vi "HFRR ADV v037 new software.vi"() -> ()   [LabVIEW 2025] (continued)
              disable-tunnel: "Heater On" -> [w1617 _]
              frame Enabled {
                n1486 = local read "EVENT LOG"() -> (w1618:string)
                n1487 = call "Event Log.vi"("Content"=w1617, "EVENT LOG"=w1618) -> ("EVENT LOG"=w1619:string)  [unwired: 8 in, 1 out]
                n1488 = local write "EVENT LOG"(w1619) -> ()
              }
              frame Disabled {
              }
            }
          }
        }
      }
    }
    n1489 = local read "Main Tab"() -> (w1340:T2)
    n1490 = case shown="\"About\"" w1340 {
      frame "HOME", Default {
        w1382 = T19."Enabled" ("Disabled")
        n1491 = local read "Service Password enable"() -> (w1384:bool)
        n1492 = property on="Imaging" class="Bool (strict)"("DisabledEnum"=w1382) -> ()  [unwired: 2 in, 2 out]
        n1493 = property on="Dashboard" class="Bool (strict)"("DisabledEnum"=w1382) -> ()  [unwired: 2 in, 2 out]
        n1494 = property on="Test Setup" class="Bool (strict)"("DisabledEnum"=w1382) -> ()  [unwired: 2 in, 2 out]
        n1495 = property on="Analysis" class="Bool (strict)"("DisabledEnum"=w1382) -> ()  [unwired: 2 in, 2 out]
        n1496 = property on="Home" class="Bool (strict)"("DisabledEnum"=w1382) -> ()  [unwired: 2 in, 2 out]
        n1497 = property on="Report" class="Bool (strict)"("DisabledEnum"=w1382) -> ()  [unwired: 2 in, 2 out]
        n1498 = property on="Main Dashboard Buttons" class="RadioBtnsControl (strict)"("DisabledEnum"=w1382) -> ()  [unwired: 2 in, 2 out]
        n1499 = property on="Calibration" class="Bool (strict)"("DisabledEnum"=w1382) -> ()  [unwired: 2 in, 2 out]
        n1500 = case shown="True" w1384 {
          tunnel: [T19."Disabled" ("Disabled") T19."Enabled" ("Disabled")] -> w1383
          frame False {
          }
          frame True {
          }
        }
        n1501 = property on="About" class="Bool (strict)"("DisabledEnum"=w1383) -> ()  [unwired: 2 in, 2 out]
      }
      frame "Test Setup" {
        w1389 = T19."Enabled" ("Disabled")
        n1502 = local read "Service Password enable"() -> (w1388:bool)
        n1503 = property on="Dashboard" class="Bool (strict)"("DisabledEnum"=T19."Disabled" ("Disabled")) -> ()  [unwired: 2 in, 2 out]
        n1504 = property on="Imaging" class="Bool (strict)"("DisabledEnum"=w1389) -> ()  [unwired: 2 in, 2 out]
        n1505 = property on="Analysis" class="Bool (strict)"("DisabledEnum"=w1389) -> ()  [unwired: 2 in, 2 out]
        n1506 = property on="Home" class="Bool (strict)"("DisabledEnum"=w1389) -> ()  [unwired: 2 in, 2 out]
        n1507 = property on="Report" class="Bool (strict)"("DisabledEnum"=w1389) -> ()  [unwired: 2 in, 2 out]
        n1508 = property on="Test Setup" class="Bool (strict)"("DisabledEnum"=w1389) -> ()  [unwired: 2 in, 2 out]
        n1509 = case shown="True" w1388 {
          tunnel: [T19."Disabled" ("Disabled") T19."Enabled" ("Disabled")] -> w1387
          frame False {
          }
          frame True {
          }
        }
        n1510 = property on="About" class="Bool (strict)"("DisabledEnum"=w1387) -> ()  [unwired: 2 in, 2 out]
      }
      frame "Adv Scar" {
        w1396 = T19."Enabled" ("Disabled")
        n1511 = property on="Dashboard" class="Bool (strict)"("DisabledEnum"=T19."Disabled" ("Disabled")) -> ()  [unwired: 2 in, 2 out]
        n1512 = property on="Imaging" class="Bool (strict)"("DisabledEnum"=w1396) -> ()  [unwired: 2 in, 2 out]
        n1513 = property on="Analysis" class="Bool (strict)"("DisabledEnum"=w1396) -> ()  [unwired: 2 in, 2 out]
        n1514 = property on="Home" class="Bool (strict)"("DisabledEnum"=w1396) -> ()  [unwired: 2 in, 2 out]
        n1515 = property on="Report" class="Bool (strict)"("DisabledEnum"=w1396) -> ()  [unwired: 2 in, 2 out]
        n1516 = property on="Test Setup" class="Bool (strict)"("DisabledEnum"=w1396) -> ()  [unwired: 2 in, 2 out]
        n1517 = local read "Service Password enable"() -> (w1394:bool)
        n1518 = case shown="True" w1394 {
          tunnel: [T19."Disabled" ("Disabled") T19."Enabled" ("Disabled")] -> w1393
          frame False {
          }
          frame True {
          }
        }
        n1519 = property on="About" class="Bool (strict)"("DisabledEnum"=w1393) -> ()  [unwired: 2 in, 2 out]
      }
      frame "Calibration" {
        w1399 = T19."Enabled" ("Disabled")
        n1520 = property on="Dashboard" class="Bool (strict)"("DisabledEnum"=T19."Disabled" ("Disabled")) -> ()  [unwired: 2 in, 2 out]
        n1521 = property on="Imaging" class="Bool (strict)"("DisabledEnum"=w1399) -> ()  [unwired: 2 in, 2 out]
        n1522 = property on="Analysis" class="Bool (strict)"("DisabledEnum"=w1399) -> ()  [unwired: 2 in, 2 out]
        n1523 = property on="Home" class="Bool (strict)"("DisabledEnum"=w1399) -> ()  [unwired: 2 in, 2 out]
        n1524 = property on="Report" class="Bool (strict)"("DisabledEnum"=w1399) -> ()  [unwired: 2 in, 2 out]
        n1525 = property on="Test Setup" class="Bool (strict)"("DisabledEnum"=w1399) -> ()  [unwired: 2 in, 2 out]
        n1526 = local read "Service Password enable"() -> (w1401:bool)
        n1527 = property on="Calibration" class="Bool (strict)"("DisabledEnum"=w1399) -> ()  [unwired: 2 in, 2 out]
        n1528 = case shown="True" w1401 {
          tunnel: [T19."Disabled" ("Disabled") T19."Enabled" ("Disabled")] -> w1400
          frame False {
          }
          frame True {
          }
        }
        n1529 = property on="About" class="Bool (strict)"("DisabledEnum"=w1400) -> ()  [unwired: 2 in, 2 out]
      }
      frame "Adv Scar Report" {
        w1407 = T19."Enabled" ("Disabled")
        n1530 = property on="Dashboard" class="Bool (strict)"("DisabledEnum"=T19."Disabled" ("Disabled")) -> ()  [unwired: 2 in, 2 out]
        n1531 = property on="Imaging" class="Bool (strict)"("DisabledEnum"=w1407) -> ()  [unwired: 2 in, 2 out]
        n1532 = property on="Analysis" class="Bool (strict)"("DisabledEnum"=w1407) -> ()  [unwired: 2 in, 2 out]
        n1533 = property on="Home" class="Bool (strict)"("DisabledEnum"=w1407) -> ()  [unwired: 2 in, 2 out]
        n1534 = property on="Report" class="Bool (strict)"("DisabledEnum"=w1407) -> ()  [unwired: 2 in, 2 out]
        n1535 = property on="Test Setup" class="Bool (strict)"("DisabledEnum"=w1407) -> ()  [unwired: 2 in, 2 out]
        n1536 = local read "Service Password enable"() -> (w1406:bool)
        n1537 = case shown="True" w1406 {
          tunnel: [T19."Disabled" ("Disabled") T19."Enabled" ("Disabled")] -> w1405
          frame False {
          }
          frame True {
          }
        }
        n1538 = property on="About" class="Bool (strict)"("DisabledEnum"=w1405) -> ()  [unwired: 2 in, 2 out]
      }
      frame "Compare Files" {
        w1413 = T19."Enabled" ("Disabled")
        n1539 = local read "Service Password enable"() -> (w1412:bool)
        n1540 = property on="Dashboard" class="Bool (strict)"("DisabledEnum"=T19."Disabled" ("Disabled")) -> ()  [unwired: 2 in, 2 out]
        n1541 = property on="Imaging" class="Bool (strict)"("DisabledEnum"=w1413) -> ()  [unwired: 2 in, 2 out]
        n1542 = property on="Analysis" class="Bool (strict)"("DisabledEnum"=w1413) -> ()  [unwired: 2 in, 2 out]
        n1543 = property on="Home" class="Bool (strict)"("DisabledEnum"=w1413) -> ()  [unwired: 2 in, 2 out]
        n1544 = property on="Report" class="Bool (strict)"("DisabledEnum"=w1413) -> ()  [unwired: 2 in, 2 out]
        n1545 = property on="Test Setup" class="Bool (strict)"("DisabledEnum"=w1413) -> ()  [unwired: 2 in, 2 out]
        n1546 = case shown="True" w1412 {
          tunnel: [T19."Disabled" ("Disabled") T19."Enabled" ("Disabled")] -> w1411
          frame False {
          }
          frame True {
          }
        }
        n1547 = property on="About" class="Bool (strict)"("DisabledEnum"=w1411) -> ()  [unwired: 2 in, 2 out]
      }
      frame "Acquire" {
        n1548 = local read "Service Password enable"() -> (w1418:bool)
        n1549 = property on="Test Setup" class="Bool (strict)"("DisabledEnum"=T19."Disabled" ("Disabled")) -> ()  [unwired: 2 in, 2 out]
        n1550 = local read "Auto Start Test"() -> (w1420:bool)
        n1551 = local read "RUN"() -> (w1422:bool)
        n1552 = case shown="True" w1418 {
          tunnel: [T19."Disabled" ("Disabled") T19."Enabled" ("Disabled")] -> w1419
          frame False {
          }
          frame True {
          }
        }
        n1553 = Or(x=w1422, y=w1420) -> (x .or. y?=w1421:bool)
        n1554 = case shown="True" w1421 {
          tunnel: [T19."Enabled" ("Disabled") T19."Disabled" ("Disabled")] -> w1417
          frame False {
          }
          frame True {
          }
        }
        n1555 = property on="About" class="Bool (strict)"("DisabledEnum"=w1419) -> ()  [unwired: 2 in, 2 out]
        n1556 = property on="Imaging" class="Bool (strict)"("DisabledEnum"=w1417) -> ()  [unwired: 2 in, 2 out]
        n1557 = property on="Dashboard" class="Bool (strict)"("DisabledEnum"=w1417) -> ()  [unwired: 2 in, 2 out]
        n1558 = property on="Analysis" class="Bool (strict)"("DisabledEnum"=w1417) -> ()  [unwired: 2 in, 2 out]
        n1559 = property on="Home" class="Bool (strict)"("DisabledEnum"=w1417) -> ()  [unwired: 2 in, 2 out]
        n1560 = property on="Report" class="Bool (strict)"("DisabledEnum"=w1417) -> ()  [unwired: 2 in, 2 out]
        n1561 = property on="Calibration" class="Bool (strict)"("DisabledEnum"=w1417) -> ()  [unwired: 2 in, 2 out]
      }
      frame "About" {
        n1562 = local read "FILE"() -> (w1436:string)
        n1563 = local read "TEST FILE NAM,E SAVED"() -> (w1429:bool)
        n1564 = call <vilib>:"Trim Whitespace.vi"("string"=w1436) -> ("trimmed string"=w1435:string)  [unwired: 1 in]
        n1565 = local read "Auto Start Test"() -> (w1439:bool)
        n1566 = String Length(string=w1435) -> (length=w1434:i32)
        n1567 = Greater?(x=w1434, y=1) -> (0:w1431:bool)
        n1568 = And(x=w1431, y=w1429) -> (x .and. y?=w1430:bool)
        n1569 = local read "RUN"() -> (w1441:bool)
        n1570 = case shown="True" w1430 {
          tunnel: [T19."Disabled" ("Disabled") T19."Enabled" ("Disabled")] -> w1432
          frame False {
          }
          frame True {
          }
        }
        n1571 = Or(x=w1441, y=w1439) -> (x .or. y?=w1440:bool)
        n1572 = property on="About" class="Bool (strict)"("DisabledEnum"=T19."Enabled" ("Disabled")) -> ()  [unwired: 2 in, 2 out]
        n1573 = case shown="False" w1440 {
          tunnel: [T19."Enabled" ("Disabled") T19."Disabled" ("Disabled")] -> w1438
          frame False {
          }
          frame True {
          }
        }
        n1574 = property on="Dashboard" class="Bool (strict)"("DisabledEnum"=w1432) -> ()  [unwired: 2 in, 2 out]
        n1575 = property on="Test Setup" class="Bool (strict)"("DisabledEnum"=T19."Disabled" ("Disabled")) -> ()  [unwired: 2 in, 2 out]
        n1576 = property on="Imaging" class="Bool (strict)"("DisabledEnum"=w1438) -> ()  [unwired: 2 in, 2 out]
        n1577 = property on="Analysis" class="Bool (strict)"("DisabledEnum"=w1438) -> ()  [unwired: 2 in, 2 out]
        n1578 = property on="Home" class="Bool (strict)"("DisabledEnum"=w1438) -> ()  [unwired: 2 in, 2 out]
        n1579 = property on="Report" class="Bool (strict)"("DisabledEnum"=w1438) -> ()  [unwired: 2 in, 2 out]
      }
    }
    n1580 = local read "Quit"() -> (w1366:bool)
    "Single" <- "Single - Graph"
  }
  n1581 = disable-structure shown="Disabled" {
    disable-tunnel: [w1719 _] -> w42
    disable-tunnel: _ -> [w1718 _]
    frame Disabled {
      n1582 = while {
        tunnel: w1718 -> [_]
        tunnel: [w1720] -> w1719
        tunnel: [w1721] -> _
        i -> [w1721]
        stop <- w1720 stop-if-true
        w1737 = u16 10 items=["1.0"=10, "1.5"=15, "2.0"=20] ("stop bits (10: 1 bit)")
        n1583 = Wait (ms)(milliseconds to wait=u32 10) -> ()  [unwired: 1 out]
        n1584 = call-poly "VISA Configure Serial Port"("VISA resource name"=refnum<visa-resource-name> "ASRL1::INSTR" ("COM PORT"), "timeout (10sec)"=u32 10, "baud rate (9600)"=u32 57600, "data bits (8)"=u16 8, "stop bits (10: 1 bit)"=w1737) -> ("VISA resource name out"=w1723:refnum<visa-resource-name>, "error out"=w1732:errorcluster)  [unwired: 9 in]
        n1585 = VISA Read(VISA resource name=w1723, byte count=u32 2 ("byte count (0)")) -> (read buffer=w1731:string)  [unwired: 1 in, 3 out]
        n1586 = String Subset(string=w1731, offset (0)=0, length (rest)=2 ("length (rest)")) -> (substring=w1730:string)
        n1587 = Match Pattern(string=w1730, regular expression="<>") -> (offset past match=w1727:i32)  [unwired: 1 in, 3 out]
        n1588 = Greater Or Equal?(x=w1727, y=0) -> (x >= y?=w1722:bool)
        n1589 = case shown="True" w1722 {
          tunnel: w1723 -> [_ w1741]
          tunnel: w1732 -> [_ w1740]
          frame False {
          }
          frame True {
            n1590 = VISA Read(VISA resource name=w1741, byte count=u32 32 ("byte count (0)"), error in (no error)=w1740) -> (read buffer=w1739:string)  [unwired: 3 out]
            n1591 = String Subset(string=w1739, offset (0)=0, length (rest)=8 ("length (rest)")) -> (substring=w1743:string)
            n1592 = String Subset(string=w1739, offset (0)=8, length (rest)=8 ("length (rest)")) -> (substring=w1744:string)
            n1593 = Decimal String To Number(string=w1744) -> (number=w1751:i32)  [unwired: 2 in, 1 out]
            n1594 = Decimal String To Number(string=w1743) -> (number=w1747:i32)  [unwired: 2 in, 1 out]
            n1595 = Divide(x=w1751, y=10000) -> ()  [unwired: 1 out]
            n1596 = Divide(x=w1747, y=1000000) -> ()  [unwired: 1 out]
          }
        }
        n1597 = local read "Quit"() -> (w1720:bool)
      }
    }
    frame Enabled {
    }
  }
  n1598 = Tick Count (ms)() -> (millisecond timer value=w4:u32)
  n1599 = while {
    shift-right: [w1797] -> _
    shift-left: w6 -> [w1801]
    shift-right: [w1796] -> _
    shift-left: w5 -> [w1800]
    shift-right: [w1795] -> _
    shift-left: w6 -> [w1799]
    shift-right: [w1794] -> _
    shift-left: w5 -> [w1798]
    shift-right: [w1792] -> _
    shift-left: w4 -> [w1793]
    shift-right: [w1789] -> _
    shift-left: w3 -> [w1790]
    shift-right: [w1788] -> _
    shift-left: w3 -> [w1791]
    shift-right: [w1781] -> _
    shift-left: w3 -> [w1787]
    shift-right: [w1780] -> _
    shift-left: w3 -> [w1786]
    shift-right: [w1779] -> _
    shift-left: w3 -> [w1785]
    shift-right: [w1778] -> _
    shift-left: w3 -> [w1784]
    shift-right: [w1777] -> _
    shift-left: w3 -> [w1783]
    shift-right: [w1776] -> _
    shift-left: w3 -> [w1782]
    shift-right: [w1775] -> _
    shift-left: w3 -> [w1769]
    shift-right: [w1774] -> _
    shift-left: w3 -> [w1768]
    shift-right: [w1773] -> _
    shift-left: w3 -> [w1767]
    shift-right: [w1772] -> _
    shift-left: w3 -> [w1766]
    shift-right: [w1771] -> _
    shift-left: w3 -> [w1765]
    shift-right: [w1770] -> _
    shift-left: w3 -> [w1764]
    shift-right: [w1755] -> _
    shift-left: w3 -> [w1758]
    shift-right: [w1754] -> _
    shift-left: w3 -> [w1757]
    shift-right: [w1753] -> _
    shift-left: w3 -> [w1756]
    stop <- w1803 stop-if-true
    n1600 = local read "Read UNO"() -> (w1762:string)
    n1601 = local read "Error  2"() -> (w1802:errorcluster)
    n1602 = String Length(string=w1762) -> (length=w1761:i32)
    n1603 = call <vilib>:"Trim Whitespace.vi"("string"=w1762) -> ("trimmed string"=w1763:string)  [unwired: 1 in]
    n1604 = Greater Or Equal?(x=w1761, y=23) -> (x >= y?=w1759:bool)
    n1605 = case shown="No Error" w1802 {
      tunnel: w1801 -> [w1849 w1945]
      tunnel: w1800 -> [w1848 w1944]
      tunnel: w1799 -> [w1847 w1943]
      tunnel: w1798 -> [w1846 w1942]
      tunnel: [w1845 w1945] -> w1797
      tunnel: [w1844 w1944] -> w1796
      tunnel: [w1843 w1943] -> w1795
      tunnel: [w1842 w1942] -> w1794
      tunnel: w1793 -> [w1841 w1941]
      tunnel: [w1840 w1941] -> w1792
      tunnel: w1790 -> [w1839 w1940]
      tunnel: w1791 -> [w1838 w1939]
      tunnel: [w1837 w1940] -> w1789
      tunnel: [w1836 w1939] -> w1788
      tunnel: w1787 -> [w1835 w1938]
      tunnel: w1786 -> [w1834 w1937]
      tunnel: w1785 -> [w1833 w1936]
      tunnel: w1784 -> [w1832 w1935]
      tunnel: w1783 -> [w1831 w1934]
      tunnel: w1782 -> [w1830 w1933]
      tunnel: [w1829 w1938] -> w1781
      tunnel: [w1828 w1937] -> w1780
      tunnel: [w1827 w1936] -> w1779
      tunnel: [w1826 w1935] -> w1778
      tunnel: [w1825 w1934] -> w1777
      tunnel: [w1824 w1933] -> w1776
      tunnel: w1769 -> [w1823 w1932]
      tunnel: [w1822 w1932] -> w1775
      tunnel: [w1821 w1928] -> w1774
      tunnel: [w1820 w1927] -> w1773
      tunnel: [w1819 w1931] -> w1772
      tunnel: [w1818 w1930] -> w1771
      tunnel: [w1817 w1929] -> w1770
      tunnel: w1768 -> [w1816 w1931]
      tunnel: w1767 -> [w1815 w1930]
      tunnel: w1766 -> [w1814 w1929]
      tunnel: w1765 -> [w1813 w1928]
      tunnel: w1764 -> [w1812 w1927]
      tunnel: w1763 -> [w1811 _]
      tunnel: w1759 -> [w1810 _]
      tunnel: w1758 -> [w1809 w1926]
      tunnel: w1757 -> [w1808 w1925]
      tunnel: w1756 -> [w1807 w1924]
      tunnel: [w1806 w1926] -> w1755
      tunnel: [w1805 w1925] -> w1754
      tunnel: [w1804 w1924] -> w1753
      frame No Error {
        n1606 = case shown="True" w1810 {
          tunnel: w1849 -> [w1865 w1917]
          tunnel: w1848 -> [w1864 w1916]
          tunnel: w1847 -> [w1863 w1915]
          tunnel: w1846 -> [w1862 w1914]
          tunnel: [w1865 w1913] -> w1845
          tunnel: [w1864 w1912] -> w1844
          tunnel: [w1863 w1911] -> w1843
          tunnel: [w1862 w1910] -> w1842
          tunnel: w1841 -> [w1861 w1908]
          tunnel: [w1861 w1907] -> w1840
          tunnel: w1839 -> [w1860 w1906]
          tunnel: w1838 -> [w1859 w1905]
          tunnel: [w1860 w1904] -> w1837
          tunnel: [w1859 w1903] -> w1836
          tunnel: w1835 -> [w1858 w1902]
          tunnel: w1834 -> [w1857 w1901]
          tunnel: w1833 -> [w1856 w1900]
          tunnel: w1832 -> [w1855 w1899]
          tunnel: w1831 -> [w1854 w1898]
          tunnel: w1830 -> [w1853 w1897]
          tunnel: [w1858 w1896] -> w1829
          tunnel: [w1857 w1895] -> w1828
          tunnel: [w1856 w1894] -> w1827
          tunnel: [w1855 w1893] -> w1826
          tunnel: [w1854 w1892] -> w1825
          tunnel: [w1853 w1891] -> w1824
          tunnel: w1823 -> [w1871 w1890]
          tunnel: [w1871 w1889] -> w1822
          tunnel: [w1868 w1888] -> w1821
          tunnel: [w1867 w1887] -> w1820
          tunnel: [w1870 w1886] -> w1819
          tunnel: [w1866 w1885] -> w1818
          tunnel: [w1869 w1884] -> w1817
          tunnel: w1816 -> [w1870 w1883]
          tunnel: w1815 -> [w1869 w1882]
          tunnel: w1814 -> [w1868 w1881]
          tunnel: w1813 -> [w1867 w1880]
          tunnel: w1812 -> [w1866 w1879]
          tunnel: w1811 -> [_ w1878]
          tunnel: w1809 -> [w1852 w1877]
          tunnel: w1808 -> [w1851 w1876]
          tunnel: w1807 -> [w1850 w1875]
          tunnel: [w1852 w1874] -> w1806
          tunnel: [w1851 w1873] -> w1805
          tunnel: [w1850 w1872] -> w1804
          frame False {
          }
          frame True {
            n1607 = Tick Count (ms)() -> (millisecond timer value=w1909:u32)
            n1608 = String To Byte Array(string=w1878) -> (unsigned byte array=w1922:u8[])
            n1609 = Array Size(array=w1922) -> (size(s)=w1921:i32)
            n1610 = formula code="// --- INTERNAL VARIABLE DECLARATIONS ---\nint i = 0;\nint k = 0;\nint start_idx = -1;\nint end_idx = -1;\nint phase = 0;\nint sign0 = 1;\nint sign1 = 1;\nint ch0_val = 0;   \nint ch1_val = 0;   \nfloat ch0_raw = 0.0;\nfloat ch1_raw = 0.0;\nfloat temp0 = 0.0;\nfloat temp1 = 0.0;\nfloat ch0_clean = 0.0;\nfloat ch1_clean = 0.0;\n\nint valid_samples = 0; // FIX: Track if we actually parsed new data this window\nfloat max_allowed_bits = 8388607.0; // FIX: Change this to match your ADC max value\n\n// Temporal intermediate variables for calculation smoothing\nfloat raw_p2p_v = 0.0;\nfloat raw_friction = 0.0;\nfloat raw_cof = 0.0;\n\n// Temporal intermediate variables for Piezo voltage translations\nfloat piezo_min_v = 0.0;\nfloat piezo_max_v = 0.0;\n\n// Initialize output variables to current shift register states right away\nout_LVDT_Min_V = in_LVDT_Min_V;\nout_LVDT_Max_V = in_LVDT_Max_V;\nout_LVDT_P2P_V = in_LVDT_P2P_V;\nout_Piezo_P2P = in_Piezo_P2P;\nout_Friction_N = in_Friction_N;\nout_COF = in_COF;\nwindow_ready = 0;\n\n// --- STEP 1: PARSE EVERY STRING IN THE BYTE ARRAY ---\nif (array_size > 2) {\n    for (i = 0; i < array_size - 1; i++) {\n        if (raw_bytes[i] == 42) { // '*' character detected\n            start_idx = i;\n        }\n        \n        // Match standard delimiter sequence \";&\" or end window character\n        if (raw_bytes[i] == 59 && raw_bytes[i+1] == 38 && start_idx != -1) { \n            end_idx = i;\n            ch0_val = 0;\n            ch1_val = 0;\n            sign0 = 1;\n            sign1 = 1;\n            phase = 0; \n\n            for (k = start_idx + 1; k < end_idx; k++) {\n                if (raw_bytes[k] == 45) { // '-' sign\n                    if (phase == 0) sign0 = -1;\n                    else sign1 = -1;\n                }\n                else if (raw_bytes[k] == 43) { // '+' sign\n                    if (phase == 0) sign0 = 1;\n                    else sign1 = 1;\n                }\n                else if (raw_bytes[k] == 59) { // ';' delimiter\n                    phase = 1; \n                }\n                else if (raw_bytes[k] >= 48 && raw_bytes[k] <= 57) { // Numeric ASCII digits\n                    if (phase == 0) {\n                        ch0_val = (ch0_val * 10) + (raw_bytes[k] - 48);\n                    } else {\n                        ch1_val = (ch1_val * 10) + (raw_bytes[k] - 48);\n                    }\n                }\n            }\n\n            // Implicit type conversion\n            ch0_raw = ch0_val * sign0 * 1.0;\n            ch1_raw = ch1_val * sign1 * 1.0;\n\n            // FIX: Sanity check / Hard-clamping to catch sudden massive ASCII noise spikes\n            if (ch0_raw > max_allowed_bits)  ch0_raw = max_allowed_bits;\n            if (ch0_raw < -max_allowed_bits) ch0_raw = -max_allowed_bits;\n            if (ch1_raw > max_allowed_bits)  ch1_raw = max_allowed_bits;\n            if (ch1_raw < -max_allowed_bits) ch1_raw = -max_allowed_bits;\n\n            // --- STEP 2: 3-SAMPLE MEDIAN FILTER ---\n            m0_2 = m0_1; m0_1 = m0_0; m0_0 = ch0_raw;\n            float s0_0 = m0_0; float s0_1 = m0_1; float s0_2 = m0_2;\n            if (s0_0 > s0_1) { temp0 = s0_0; s0_0 = s0_1; s0_1 = temp0; }\n            if (s0_1 > s0_2) { temp0 = s0_1; s0_1 = s0_2; s0_2 = temp0; }\n            if (s0_0 > s0_1) { temp0 = s0_0; s0_0 = s0_1; s0_1 = temp0; }\n            ch0_clean = s0_1;\n\n            m1_2 = m1_1; m1_1 = m1_0; m1_0 = ch1_raw;\n            float s1_0 = m1_0; float s1_1 = m1_1; float s1_2 = m1_2;\n            if (s1_0 > s1_1) { temp1 = s1_0; s1_0 = s1_1; s1_1 = temp1; }\n            if (s1_1 > s1_2) { temp1 = s1_1; s1_1 = s1_2; s1_2 = temp1; }\n            if (s1_0 > s1_1) { temp1 = s1_0; s1_0 = s1_1; s1_1 = temp1; }\n            ch1_clean = s1_1;\n\n            // --- STEP 3: EXPONENTIAL FILTER (STREAM LEVEL) ---\n            if (ch0_filt == 0.0) ch0_filt = ch0_clean;\n            if (ch1_filt == 0.0) ch1_filt = ch1_clean;\n\n            ch0_filt = ch0_filt + (ch0_clean - ch0_filt) * 0.125;\n            ch1_filt = ch1_filt + (ch1_clean - ch1_filt) * 0.125;\n\n            // --- STEP 4: MIN/MAX WINDOW CONTINUOUS ACCUMULATION ---\n            if (ch0_filt > max_ch0) max_ch0 = ch0_filt;\n            if (ch0_filt < min_ch0) min_ch0 = ch0_filt;\n            if (ch1_filt > max_ch1) max_ch1 = ch1_filt;\n            if (ch1_filt < min_ch1) min_ch1 = ch1_filt;\n\n            valid_samples++; // FIX: Successfully parsed and accumulated a clean point\n            start_idx = -1; \n        }\n    }\n}\n\n// --- STEP 5: WINDOW EVALUATION ENGINE ---\n// FIX: Condition updated to verify that valid samples exist for both channels\nif (((current_time_ms - start_time_ms) >= 50) && (valid_samples > 0) && (min_ch0 < 9000000.0) && (min_ch1 < 9000000.0)) {\n    window_ready = 1;\n\n    // Linear Bit-to-Voltage Transformations (LVDT - Channel 0)\n    out_LVDT_Min_V = (min_ch0 * VREF) / 8388607.0;\n    out_LVDT_Max_V = (max_ch0 * VREF) / 8388607.0;\n    raw_p2p_v = out_LVDT_Max_V - out_LVDT_Min_V;\n\n    // Linear Bit-to-Voltage Transformations (Piezo - Channel 1)\n    piezo_min_v = (min_ch1 * VREF) / 8388607.0;\n    piezo_max_v = (max_ch1 * VREF) / 8388607.0;\n    \n    // Assign Peak-to-Peak Voltage directly to output indicator (Matches Python logic)\n    out_Piezo_P2P = piezo_max_v - piezo_min_v;\n    \n    // Force scaling calculations using Voltage delta * Newtons/Volt Factor\n    raw_friction = out_Piezo_P2P * PIEZO_CAL_FACTOR + 0.44528;\n    raw_cof = raw_friction / NORMAL_FORCE;\n\n    // --- STEP 6: OUTPUT METRIC SMOOTHING (Low-Pass Filter Alpha = 0.05) ---\n    // Seed initial historical metrics if first loop iteration\n    if (hist_LVDT_P2P == 0.0) hist_LVDT_P2P = raw_p2p_v;\n    if (hist_Friction == 0.0) hist_Friction = raw_friction;\n    if (hist_COF == 0.0)      hist_COF = raw_cof;\n\n    // Apply exponential output dampening\n    hist_LVDT_P2P = hist_LVDT_P2P + (raw_p2p_v - hist_LVDT_P2P) * 0.05;\n    hist_Friction = hist_Friction + (raw_friction - hist_Friction) * 0.05; // Note: Can drop to 0.02 for more aggressive damping\n    hist_COF      = hist_COF + (raw_cof - hist_COF) * 0.05;\n\n    // Direct smoothed parameters out to UI Indicators\n    out_LVDT_P2P_V = hist_LVDT_P2P;\n    out_Friction_N = hist_Friction;\n    out_COF        = hist_COF;\n\n    // Reset tracking targets to extreme boundaries safely\n    min_ch0 = 9999999.0;\n    max_ch0 = -9999999.0;\n    min_ch1 = 9999999.0;\n    max_ch1 = -9999999.0;\n\n    valid_samples = 0; // FIX: Reset counter for next time frame\n    start_time_ms = current_time_ms;\n}"("raw_bytes"=w1922, "array_size"=w1921, "VREF"="VREF", "PIEZO_CAL_FACTOR"="PIEZO_CAL_FACTOR", "NORMAL_FORCE"="NORMAL_FORCE", "min_ch0"=w1917, "max_ch0"=w1916, "min_ch1"=w1915, "max_ch1"=w1914, "current_time_ms"=w1909, "start_time_ms"=w1908, "ch0_filt"=w1906, "ch1_filt"=w1905, "m0_0"=w1902, "m0_1"=w1901, "m0_2"=w1900, "m1_0"=w1899, "m1_1"=w1898, "m1_2"=w1897, "in_LVDT_Min_V"=w1890, "in_LVDT_Max_V"=w1883, "in_LVDT_P2P_V"=w1882, "in_Piezo_P2P"=w1881, "in_Friction_N"=w1880, "in_COF"=w1879, "hist_LVDT_P2P"=w1877, "hist_Friction"=w1876, "hist_COF"=w1875) -> ("window_ready"=→"Valid_data":dbl, "out_LVDT_Min_V"=w1889:dbl, "out_LVDT_Max_V"=w1888:dbl, "out_LVDT_P2P_V"=w1887:dbl, "out_Piezo_P2P"=w1886:dbl, "out_Friction_N"=w1885:dbl, "out_COF"=w1884:dbl, "min_ch0"=w1913:dbl, "max_ch0"=w1912:dbl, "min_ch1"=w1911:dbl, "max_ch1"=w1910:dbl, "start_time_ms"=w1907:u32, "ch0_filt"=w1904:dbl, "ch1_filt"=w1903:dbl, "m0_0"=w1896:dbl, "m0_1"=w1895:dbl, "m0_2"=w1894:dbl, "m1_0"=w1893:dbl, "m1_1"=w1892:dbl, "m1_2"=w1891:dbl, "hist_LVDT_P2P"=w1874:dbl, "hist_Friction"=w1873:dbl, "hist_COF"=w1872:dbl)
            "LVDT MIN" <- w1889
            "LVDT MAX" <- w1888
            "LVDT Peak" <- w1887
            "pizo raw" <- w1886
            "cof" <- w1884
            "Frictioin Force Raw" <- w1885
          }
        }
      }
      frame Error {
      }
    }
    n1611 = local read "Quit"() -> (w1803:bool)
  }
  n1612 = disable-structure shown="Disabled" {
    disable-tunnel: errorcluster {"status"=TRUE, "code"=0, "source"="Init"} ("error IO") -> [w1948 _]
    disable-tunnel: [w1946 _] -> w45
    frame Disabled {
      n1613 = while {
        shift-right: [w1964] -> w1950
        shift-left: _ -> [w1955]
        shift-right: [w1963] -> w1949
        shift-left: w1948 -> [w1957]
        tunnel: [w1952] -> w1946
        tunnel: [w1962] -> _
        i -> [w1962]
        stop <- w1952 stop-if-true
        n1614 = local read "Port 1a"() -> (w1958:bool)
        n1615 = local read "Port 3"() -> (w1959:bool)
        n1616 = local read "Com Port 1"() -> (w1956:refnum<visa-resource-name>)
        n1617 = Or(x=w1959, y=w1958) -> (x .or. y?=w1961:bool)
        n1618 = Unbundle(w1957) -> ("status"=→"Port 3":bool)  [unwired: 2 out]
        n1619 = Not Equal?(x=w1956, y=w1955) -> (x != y?=w1953:bool)
        n1620 = case shown="True" w1961 {
          frame False {
            w1967 = TRUE ("Visible")
            n1621 = property on="Port 1a" class="Bool (strict)"("Visible"=w1967) -> ()  [unwired: 2 in, 2 out]
            n1622 = property on="Port 3" class="Bool (strict)"("Visible"=w1967) -> ()  [unwired: 2 in, 2 out]
          }
          frame True {
            w1968 = TRUE ("Visible")
            n1623 = property on="Port 1a" class="Bool (strict)"("Visible"=w1968) -> ()  [unwired: 2 in, 2 out]
            n1624 = property on="Port 3" class="Bool (strict)"("Visible"=w1968) -> ()  [unwired: 2 in, 2 out]
          }
        }
        n1625 = Wait (ms)(milliseconds to wait=u32 40) -> ()  [unwired: 1 out]
        n1626 = case shown="True" w1953 {
          tunnel: [w1965 errorcluster {"status"=TRUE, "code"=0, "source"="Init"} ("error out")] -> w1954
          tunnel: w1957 -> [w1965 _]
          frame False {
          }
          frame True {
          }
        }
        n1627 = case shown="Error" w1954 {
          selector: w1954 -> [w1975 w1993]
          tunnel: [w1978 w1997] -> w1964
          tunnel: [w1977 w1991] -> w1963
          tunnel: w1955 -> [w1976 w1995]
          frame No Error {
            n1628 = property class="Instr"(reference=w1976, error in=w1975) -> (reference out=w1973:refnum<visa-resource-name>, error out=w1974:errorcluster, "Serial Settings:Number of Bytes at Serial Port"=w1970:u32)
            n1629 = Greater?(x=w1970, y=u32 5) -> (0:w1969:bool)
            n1630 = Not(x=w1969) -> (.not. x?=→"Port 1a":bool)
            n1631 = while {
              tunnel: [w1986] -> w1977
              tunnel: [w1985] -> w1978
              tunnel: w1974 -> [w1984]
              tunnel: w1973 -> [w1983]
              stop <- TRUE stop-if-true
              n1632 = property class="Instr" props=["Serial Settings:Number of Bytes at Serial Port"](reference=w1983, error in=w1984) -> (reference out=w1988:refnum<visa-resource-name>, error out=w1987:errorcluster)  [unwired: 1 out]
              n1633 = VISA Read(VISA resource name=w1988, byte count=u32 50, error in (no error)=w1987) -> (VISA resource name out=w1985:refnum<visa-resource-name>, read buffer=w1980:string, error out=w1986:errorcluster)  [unwired: 1 out]
              n1634 = Wait (ms)(milliseconds to wait=u32 5) -> ()  [unwired: 1 out]
            }
          }
          frame Error {
            w2003 = u16 0 items=["None", "XON/XOFF", "RTS/CTS", "XON/XOFF & RTS/CTS", "DTR/DSR", "XON/XOFF & DTR/DSR"] ("flow control (0:none)  2")
            w2001 = u16 10 items=["1.0"=10, "1.5"=15, "2.0"=20] ("stop bits 2")
            w1999 = u16 0 items=["None", "Odd", "Even", "Mark", "Space"] ("parity 2")
            w2000 = u32 10000  # timeout (10sec)
            n1635 = VISA Close(VISA resource name=w1995, error in (no error)=w1993) -> (error out=w1996:errorcluster)
            n1636 = local write "Port 1a"(FALSE ("Port 1a")) -> ()
            n1637 = local read "Com Port 1"() -> (w1990:refnum<visa-resource-name>)
            n1638 = call <vilib>:"Clear Errors.vi"("error in (no error)"=w1996) -> ("error out"=w1994:errorcluster)  [unwired: 5 in, 1 out]
            n1639 = call-poly "VISA Configure Serial Port"("VISA resource name"=w1990, "timeout (10sec)"=w2000, "baud rate (9600)"=u32 250000 ("baud rate  2"), "data bits (8)"=u16 8 ("data bits  2"), "parity (0:none)"=w1999, "error in (no error)"=w1994, "stop bits (10: 1 bit)"=w2001, "flow control (0:none)"=w2003) -> ("VISA resource name out"=w2004:refnum<visa-resource-name>, "error out"=w2005:errorcluster)  [unwired: 6 in]
            n1640 = flat-sequence {
              tunnel: w2004 -> [w2007]
              tunnel: w2005 -> [w2006]
              tunnel: [w2007] -> w1997
              tunnel: [w2006] -> w1991
              frame #0 {
                n1641 = Wait (ms)(milliseconds to wait=u32 50) -> ()  [unwired: 1 out]
              }
            }
            "Residual Uno" <- ""
          }
        }
        n1642 = local read "Quit"() -> (w1952:bool)
        "Error Uno" <- w1957
      }
      n1643 = VISA Close(VISA resource name=w1950, error in (no error)=w1949) -> (error out=w1947:errorcluster)
      n1644 = call <vilib>:"Clear Errors.vi"("error in (no error)"=w1947) -> ()  [unwired: 5 in, 2 out]
    }
    frame Enabled {
    }
  }
  n1645 = while {
    stop <- w2018 stop-if-true
    # "V0OLTAGE TO STROKE (peice vise calibration)"
    n1646 = local read "LVDT MIN"() -> (w2010:dbl)
    n1647 = local read "LVDT Peak"() -> (w2009:dbl)
    n1648 = Wait (ms)(milliseconds to wait=u32 10) -> ()  [unwired: 1 out]
    n1649 = formula code="// Dynamic Parameterized Linear Interpolation Node\n// Inputs: vpp_val, voltages (Array), distances (Array)\n// Outputs: stroke\n\nint i = 0;\nint segments = 11; // 12 points make 11 interpolation segments\n\n// 1. Lower Boundary Clamp\nif (vpp_val <= voltages[0]) {\n    stroke = distances[0];\n}\n// 2. Upper Boundary Clamp\nelse if (vpp_val >= voltages[segments]) {\n    stroke = distances[segments];\n}\n// 3. Dynamic Segment Search Loop\nelse {\n    stroke = distances[0]; // Fallback baseline\n    for (i = 0; i < segments; i++) {\n        if (vpp_val >= voltages[i] && vpp_val <= voltages[i+1]) {\n            // Standard linear interpolation formula using array lookups\n            stroke = distances[i] + (vpp_val - voltages[i]) * (distances[i+1] - distances[i]) / (voltages[i+1] - voltages[i]);\n            break; // Segment found, safely exit the loop\n        }\n    }\n}"("vpp_val"=w2009, "voltages"="calibration values", "distances"="STROKE") -> ("stroke"=→"LVDT STROKE":dbl)
    n1650 = local read "Calibration Tare Value"() -> (w2014:dbl)
    n1651 = local read "Calibration Tare"() -> (w2012:bool)
    n1652 = Subtract(x=w2010, y=w2014) -> (x-y=→"LVDT STROKE  Calibration":dbl)
    n1653 = case shown="True" w2012 {
      selector: w2012 -> [_ w2020]
      tunnel: w2010 -> [_ w2021]
      frame False {
      }
      frame True {
        n1654 = Not(x=w2020) -> (.not. x?=w2019:bool)
        n1655 = local write "Calibration Tare"(w2019) -> ()
        "Calibration Tare Value" <- w2021
      }
    }
    n1656 = local read "Quit"() -> (w2018:bool)
  }
  n1657 = while {
    stop <- w2044 stop-if-true
    n1658 = local read "Due read"() -> (w2042:string)
    n1659 = call <vilib>:"High Resolution Polling Wait.vi"("seconds to wait"=0.02) -> ()  [unwired: 10 in, 1 out]
    n1660 = local read "Frictioin Force Raw"() -> (w2024:dbl)
    n1661 = Spreadsheet String To Array(delimiter (Tab)=";", format string="", spreadsheet string=w2042, array type (2D Dbl)=string[] []) -> (array=w2039:string[])
    n1662 = Fract/Exp String To Number(string=w2039) -> (number=w2038:dbl[])  [unwired: 3 in, 1 out]
    n1663 = call <vilib>:"Median Filter PtByPt.vi"("rank"=2, "x"=w2024) -> ("Filtered x"=→"Friction":dbl)  [unwired: 2 in, 1 out]
    n1664 = Index Array(array=w2038) -> (element #1=→"Sample Temperature":dbl, element #2=→"Target Sample Temperature":dbl, element #3=→"Current Duty Cycle":dbl, element #4=→"Ambient Temperature":dbl, element #5=→"Dac Status":dbl, element #6=→"Vpp":dbl, element #7=→"Active Error Code":dbl, element #8=→"Kp":dbl, element #9=→"Ki":dbl, element #10=→"Kd":dbl, element #11=→"SampleRaw":dbl, element #12=→"AmbRaw":dbl)  [unwired: 12 in]
    n1665 = local read "Quit"() -> (w2044:bool)
  }
  n1666 = while {
    shift-right: [w2058] -> w41
    shift-left: _ -> [w2050]
    shift-right: [w2045] -> w40
    shift-left: errorcluster {"status"=FALSE, "code"=0, "source"="Init"} ("error out") -> [w2052]
    tunnel: [w2047] -> w44
    tunnel: [w2057] -> _
    i -> [w2057]
    stop <- w2047 stop-if-true
    n1667 = local read "Com Port 2"() -> (w2051:refnum<visa-resource-name>)
    n1668 = local read "Port 2a"() -> (w2053:bool)
    n1669 = Unbundle(w2052) -> ("status"=→"Port 4":bool)  [unwired: 2 out]
    n1670 = call <vilib>:"High Resolution Polling Wait.vi"("seconds to wait"=0.02) -> ()  [unwired: 10 in, 1 out]
    n1671 = local read "Port 4"() -> (w2054:bool)
    n1672 = Not Equal?(x=w2051, y=w2050) -> (x != y?=w2049:bool)
    n1673 = Or(x=w2054, y=w2053) -> (x .or. y?=w2056:bool)
    n1674 = case shown="False" w2056 {
      frame False {
        w2061 = TRUE ("Visible")
        n1675 = property on="Port 2a" class="Bool (strict)"("Visible"=w2061) -> ()  [unwired: 2 in, 2 out]
        n1676 = property on="Port 4" class="Bool (strict)"("Visible"=w2061) -> ()  [unwired: 2 in, 2 out]
      }
      frame True {
        w2062 = TRUE ("Visible")
        n1677 = property on="Port 2a" class="Bool (strict)"("Visible"=w2062) -> ()  [unwired: 2 in, 2 out]
        n1678 = property on="Port 4" class="Bool (strict)"("Visible"=w2062) -> ()  [unwired: 2 in, 2 out]
      }
    }
    n1679 = case shown="True" w2049 {
      tunnel: [w2059 errorcluster {"status"=TRUE, "code"=0, "source"="Init"} ("error out")] -> w2048
      tunnel: w2052 -> [w2059 _]
      frame False {
      }
      frame True {
      }
    }
    n1680 = case shown="No Error" w2048 {
      selector: w2048 -> [w2075 w2106]
      tunnel: [w2068 w2111] -> w2058
      tunnel: [w2076 w2104] -> w2045
      tunnel: w2050 -> [w2077 w2109]
      frame No Error {
        n1681 = property class="Instr" props=["Serial Settings:Number of Bytes at Serial Port"](reference=w2077, error in=w2075) -> (reference out=w2069:refnum<visa-resource-name>, error out=w2074:errorcluster)  [unwired: 1 out]
        n1682 = while {
          tunnel: [w2085] -> w2070
          tunnel: [w2084] -> w2071
          tunnel: w2074 -> [w2083]
          tunnel: w2069 -> [w2082]
          tunnel: [w2081] -> _
          i -> [w2081]
          stop <- TRUE stop-if-true
          n1683 = property class="Instr" props=["Serial Settings:Number of Bytes at Serial Port"](reference=w2082, error in=w2083) -> (reference out=w2087:refnum<visa-resource-name>, error out=w2086:errorcluster)  [unwired: 1 out]
          n1684 = VISA Read(VISA resource name=w2087, byte count=u32 1000, error in (no error)=w2086) -> (VISA resource name out=w2084:refnum<visa-resource-name>, read buffer=→"Due read":string, error out=w2085:errorcluster)  [unwired: 1 out]
        }
        n1685 = local read "Due Write"() -> (w2067:string)
        n1686 = call <vilib>:"Trim Whitespace.vi"("string"=w2067) -> ("trimmed string"=w2066:string)  [unwired: 1 in]
        n1687 = Not Equal?(x=w2066, y="") -> (x != y?=w2072:bool)
        n1688 = VISA Flush I/O Buffer(VISA resource name=w2071) -> (VISA resource name out=w2064:refnum<visa-resource-name>, error out=→"error out 10":errorcluster)  [unwired: 2 in]
        n1689 = case shown="True" w2072 {
          tunnel: w2064 -> [w2089 w2094]
          tunnel: [w2089 w2098] -> w2068
          tunnel: w2070 -> [w2088 w2093]
          tunnel: [w2088 w2096] -> w2076
          tunnel: w2066 -> [_ w2092]
          tunnel: [_ w2095] -> _
          frame False {
            # "DATA  WRITE LOOP"
          }
          frame True {
            n1690 = Concatenate Strings(w2092, "\r\n") -> (w2091:string)
            n1691 = VISA Write(VISA resource name=w2094, write buffer=w2091, error in (no error)=w2093) -> (VISA resource name out=w2098:refnum<visa-resource-name>, return count=w2095:u32, error out=w2097:errorcluster)
            n1692 = flat-sequence {
              tunnel: w2097 -> [w2100]
              tunnel: [w2100] -> w2096
              frame #0 {
                n1693 = local write "Due Write"("" ("Command")) -> ()
                n1694 = Wait (ms)(milliseconds to wait=u32 5) -> ()  [unwired: 1 out]
              }
            }
          }
        }
        "Port 2a" <- TRUE ("Port 2a")
      }
      frame Error {
        w2117 = u16 0 items=["None", "XON/XOFF", "RTS/CTS", "XON/XOFF & RTS/CTS", "DTR/DSR", "XON/XOFF & DTR/DSR"] ("flow control (0:none)  2")
        w2115 = u16 10 items=["1.0"=10, "1.5"=15, "2.0"=20] ("stop bits 2")
        w2113 = u16 0 items=["None", "Odd", "Even", "Mark", "Space"] ("parity 2")
        w2114 = u32 10000  # timeout (10sec)
        n1695 = VISA Clear(VISA resource name=w2109, error in (no error)=w2106) -> (VISA resource name out=w2108:refnum<visa-resource-name>, error out=w2107:errorcluster)
        n1696 = VISA Close(VISA resource name=w2108, error in (no error)=w2107) -> (error out=w2110:errorcluster)
        n1697 = call <vilib>:"Clear Errors.vi"("error in (no error)"=w2110) -> ()  [unwired: 5 in, 2 out]
        n1698 = local write "Port 2a"(FALSE ("Port 2a")) -> ()
        n1699 = local read "Com Port 2"() -> (w2103:refnum<visa-resource-name>)
        "visa due" <- w2103
        n1700 = call-poly "VISA Configure Serial Port"("VISA resource name"=w2103, "timeout (10sec)"=w2114, "baud rate (9600)"=u32 250000 ("baud rate  2"), "data bits (8)"=u16 8 ("data bits  2"), "parity (0:none)"=w2113, "stop bits (10: 1 bit)"=w2115, "flow control (0:none)"=w2117) -> ("VISA resource name out"=w2118:refnum<visa-resource-name>, "error out"=w2119:errorcluster)  [unwired: 7 in]
        n1701 = flat-sequence {
          tunnel: w2118 -> [w2121]
          tunnel: w2119 -> [w2120]
          tunnel: [w2121] -> w2111
          tunnel: [w2120] -> w2104
          frame #0 {
            n1702 = Wait (ms)(milliseconds to wait=u32 50) -> ()  [unwired: 1 out]
          }
        }
        "Residual Due" <- ""
      }
    }
    "error out 9" <- w2045
    n1703 = local read "Quit"() -> (w2047:bool)
    "Error Due" <- w2052
  }
  n1704 = local write "FRICVALZ"(0.0 ("FRICVALZ")) -> ()
  n1705 = property on="RUN" class="Bool (strict)"("Visible"=TRUE) -> ()  [unwired: 2 in, 2 out]
  n1706 = while {
    tunnel: [w2136] -> _
    tunnel: [w2123] -> w54
    i -> [w2136]
    stop <- w2123 stop-if-true
    n1707 = local read "conststatus"() -> (w2127:dbl)
    n1708 = local read "Main Tab"() -> (w2125:T2)
    n1709 = local read "EDIT"() -> (w2142:bool)
    n1710 = local read "Rate"() -> (w2141:dbl)
    n1711 = case shown="True" w2142 {
      tunnel: [FALSE TRUE] -> _
      frame False {
      }
      frame True {
      }
    }
    n1712 = Equal?(x=w2125, y=T28."About" ("Main Tab")) -> (x = y?=w2134:bool)
    n1713 = Equal?(x=w2127, y=0.0) -> (x = y?=w2128:bool)
    n1714 = Divide(x=1.0, y=w2141) -> (x/y=w2137:dbl)
    "Time 2" <- w2137
    n1715 = case shown="True" w2128 {
      frame False {
      }
      frame True {
        # "C:\\WinDucom\\calibrate WO 2391.dcf"
        n1716 = local write "Lan flag"(22) -> ()
        n1717 = local write "conststatus"(10.0 ("rpm value : 2")) -> ()
        n1718 = String To Path(string="C:\\LAB-IQ\\calibrate WO 2465.dcf") -> (path=w2148:path)
        n1719 = Open/Create/Replace File "Open File"(file path (use dialog)=w2148) -> (refnum out=w2146:refnum<file>)  [unwired: 5 in, 2 out]
        n1720 = for {
          N: 23 -> [_]
          tunnel: w2146 -> [w2157]
          i -> [w2151]
          (unwired) TRUE ("line mode (F)")
          n1721 = Read from Text File "Read File"(file (use dialog)=w2157) -> (text=w2156:string)  [unwired: 3 in, 3 out]
          n1722 = Match Pattern(string=w2156, regular expression="]") -> (after substring=w2154:string)  [unwired: 1 in, 3 out]
          n1723 = String Subset(string=w2156, offset (0)=5, length (rest)=10 ("length (rest)")) -> (substring=w2149:string)
          n1724 = Fract/Exp String To Number(string=w2149) -> (number=w2150:dbl)  [unwired: 3 in, 1 out]
          n1725 = Match Pattern(string=w2154, regular expression="-") -> (before substring=w2152:string)  [unwired: 1 in, 3 out]
          n1726 = case shown="10" w2151 {
            tunnel: w2150 -> [_ _ _ _ _ _ _ _ _ _ w2164 _ _ _ _ _ _ _ _ _ _ _ _ _]
            tunnel: w2152 -> [_ _ _ _ w2160 w2161 w2162 _ _ _ _ _ _ _ _ _ _ _ _ _ w2165 w2166 w2167 _]
            frame 0 {
            }
            frame 1 {
            }
            frame 2 {
            }
            frame 3 {
            }
            frame 4 {
              n1727 = local write "Com Port 1"(w2160) -> ()
            }
            frame 5 {
              n1728 = local write "Com Port 2"(w2161) -> ()
              n1729 = local write "visa due"(w2161) -> ()
            }
            frame 6 {
              n1730 = String To Path(string=w2162) -> (path=w2163:path)
              n1731 = local write "File Path"(w2163) -> ()
              "String" <- w2162
            }
            frame 7 {
            }
            frame 8 {
            }
            frame 9 {
            }
            frame 10 {
              n1732 = local write "Language Selection"(w2164) -> ()
            }
            frame 11 {
            }
            frame 12 {
            }
            frame 13 {
            }
            frame 14 {
            }
            frame 15 {
            }
            frame 16 {
            }
            frame 17 {
            }
            frame 18 {
            }
            frame 21 {
            }
            frame 22 {
              n1733 = local write "Com Port 3"(w2165) -> ()
            }
            frame 20 {
              n1734 = local write "Camera Port :"(w2166) -> ()
            }
            frame 19 {
              n1735 = local write "C3 :"(w2167) -> ()
            }
            frame 23, Default {
            }
          }
        }
      }
    }
    n1736 = Select(t=u32 2500 ("milliseconds to wait"), s=w2134, f=u32 500 ("milliseconds to wait")) -> (s? t:f=w2132:u32)
    n1737 = Multiply(x=w2137, y=w2132) -> (x*y=w2139:dbl)
    n1738 = call "Elapsed Time2"("Time Target (s)"=w2139, "Auto Reset"=TRUE) -> ("Time has Elapsed"=w2129:bool)  [unwired: 10 in, 7 out]
    n1739 = case shown="True" w2129 {
      frame False {
      }
      frame True {
        n1740 = stacked-sequence {
          frame #0 {
            # "DATA PROCESSING"
            # "115 mV/N"
            n1741 = local read "Sample Temperature"() -> (w2170:dbl)
            n1742 = local read "RH Numeric:"() -> (→"Humidity ( %RH )" →"Hum":dbl)
            n1743 = local read "FRICVALZ"() -> (w2187:dbl)
            n1744 = local read "Friction"() -> (w2173:dbl)
            n1745 = call <vilib>:"Mean PtByPt.vi"("x"=w2170, "sample length"=100) -> ("mean"=w2169:dbl)  [unwired: 2 in, 1 out]
            "TEMP 2" <- w2169
            "TEMP 3" <- w2169
            n1746 = Subtract(x=w2173, y=w2187) -> (x-y=w2182:dbl)
            "FF 2" <- w2182
            "FF 4" <- w2182
            n1747 = local read "Ambient Temperature"() -> (→"AIR TEMP":dbl)
            n1748 = local read "TEMP"() -> (w2186:dbl)
            n1749 = local write "FF 3"(w2182) -> ()
            n1750 = Compound Arithmetic op=OR("FRICVALZ 4", "FRICVALZ 3", "FRICVALZ 2") -> (w2178:bool)
            n1751 = case shown="True" w2178 {
              tunnel: w2173 -> [_ w2193]
              frame False {
              }
              frame True {
                w2192 = FALSE ("FRICVALZ")
                n1752 = local write "FRICVALZ 3"(w2192) -> ()
                n1753 = local write "FRICVALZ 2"(w2192) -> ()
                n1754 = local write "FRICVALZ 4"(w2192) -> ()
                "FRICVALZ" <- w2193
              }
            }
            n1755 = Not A Number/Path/Refnum?(number/path/refnum=w2186) -> (NaN/Path/Refnum?=w2185:bool)
            n1756 = Not A Number/Path/Refnum?(number/path/refnum=w2182) -> (NaN/Path/Refnum?=w2184:bool)
            n1757 = Divide(x=w2182, y=1.96) -> (x/y=w2179:dbl)
            n1758 = Compound Arithmetic op=OR(w2185, w2184) -> (w2183:bool)
            n1759 = Not A Number/Path/Refnum?(number/path/refnum=w2179) -> (NaN/Path/Refnum?=w2180:bool)
            n1760 = case shown="True" w2183 {
              frame False {
              }
              frame True {
                n1761 = local write "TEMP"(0.0 ("TEMP")) -> ()
                n1762 = local write "FF 2"(0.0 ("FF 2")) -> ()
                n1763 = local write "reinit"(TRUE ("reinit")) -> ()
              }
            }
            n1764 = local write "TEMP"(w2169) -> ()
            n1765 = Select(t=0.0, s=w2180, f=w2179) -> (s? t:f=w2172:dbl)
            "COF 2" <- w2172
            n1766 = local write "COF 3"(w2172) -> ()
          }
        }
      }
    }
    n1767 = Wait (ms)(milliseconds to wait=u32 50) -> ()  [unwired: 1 out]
    n1768 = local read "Quit"() -> (w2123:bool)
    "Rate" <- 2500.0 ("No of Samples")
  }
  n1769 = while {
    tunnel: [w2213] -> _
    tunnel: [w2196] -> w56
    tunnel: w1 -> [_]
    i -> [w2213]
    stop <- w2196 stop-if-true
    # "C:\\LAB-IQ-NXT\\Scar View.exe"
    n1770 = local read "OK Button 16"() -> (w2203:bool)
    n1771 = local read "Main Tab"() -> (w2197:T2)
    n1772 = local read "service 3"() -> (w2198:bool)
    n1773 = local read "OPEN 6"() -> (w2200:bool)
    n1774 = local read "EDIT 2"() -> (w2202:bool)
    n1775 = flat-sequence {
      frame #0 {
        n1776 = stacked-sequence {
          frame #0 {
            n1777 = local read "EDIT"() -> (w2691:bool)
            n1778 = case shown="False" w2691 {
              tunnel: [u8 2 ("Disabled") u8 0 ("Disabled")] -> _
              frame False {
                w2693 = FALSE
                n1779 = local write "Password"("") -> ()
                n1780 = local write "x = y?"(w2693) -> ()
                n1781 = property on="Password" class="Str"("Visible"=w2693) -> ()  [unwired: 2 in, 2 out]
              }
              frame True {
                n1782 = property on="Password" class="Str"("Visible"=TRUE) -> ()  [unwired: 2 in, 2 out]
              }
            }
            "dipl pwd" <- "@143$\n" ("dipl pwd")
          }
          frame #1 {
          }
          frame #2 {
          }
          frame #3 {
          }
          frame #4 {
            n1783 = String To Byte Array(string="Password") -> (unsigned byte array=w2704:u8[])
            n1784 = Search 1D Array(1D array=w2704, element=u8 10) -> (index of element=w2702:i32)  [unwired: 1 in]
            n1785 = Index Array(array=w2704, index=w2702) -> (element=w2703:u8)
            n1786 = Equal?(x=w2703, y=10) -> (x = y?=w2699:bool)
            n1787 = case shown="True" w2699 {
              frame False {
              }
              frame True {
                # "password"
                # "password"
                n1788 = local read "Password"() -> (w2716:string)
                n1789 = String To Byte Array(string=w2716) -> (unsigned byte array=w2719:u8[])
                n1790 = String To Byte Array(string="@143$\n") -> (unsigned byte array=w2706:u8[])
                n1791 = Array Size(array=w2719) -> (size(s)=w2715:i32)
                n1792 = Array Size(array=w2706) -> (size(s)=w2711:i32)
                n1793 = for {
                  N: w2715 -> [_]
                  tunnel: w2719 -> [w2732]
                  tunnel: [w2730] -> w2720 mode=indexing
                  tunnel: w2715 -> [w2727]
                  i -> [w2728]
                  n1794 = Decrement(x=w2727) -> (x-1=w2726:i32)
                  n1795 = Index Array(array=w2732, index=w2728) -> (element=w2731:u8)
                  n1796 = Equal?(x=w2728, y=w2726) -> (x = y?=w2725:bool)
                  n1797 = Number To Decimal String(number=w2731) -> (decimal integer string=w2729:string)  [unwired: 1 in]
                  n1798 = Select(t="", s=w2725, f="\r") -> (s? t:f=w2722:string)
                  n1799 = Concatenate Strings(w2729, w2722) -> (w2730:string)
                }
                n1800 = for {
                  N: w2711 -> [_]
                  tunnel: w2706 -> [w2743]
                  tunnel: [w2741] -> w2709 mode=indexing
                  tunnel: w2711 -> [w2738]
                  i -> [w2739]
                  n1801 = Decrement(x=w2738) -> (x-1=w2737:i32)
                  n1802 = Index Array(array=w2743, index=w2739) -> (element=w2742:u8)
                  n1803 = Equal?(x=w2739, y=w2737) -> (x = y?=w2736:bool)
                  n1804 = Number To Decimal String(number=w2742) -> (decimal integer string=w2740:string)  [unwired: 1 in]
                  n1805 = Select(t="", s=w2736, f="\r") -> (s? t:f=w2733:string)
                  n1806 = Concatenate Strings(w2740, w2733) -> (w2741:string)
                }
                n1807 = local read "file path"() -> (w2705:path)
                n1808 = call <vilib>:"Read Characters From File.vi"("file path (dialog if empty)"=w2705) -> ("character string"=w2718:string)  [unwired: 5 in, 3 out]
                "string" <- w2718
                n1809 = flat-sequence {
                  tunnel: [w2721] -> _
                  frame #0 {
                    w2721 = ""
                    n1810 = local write "Password"(w2721) -> ()
                  }
                }
                n1811 = Concatenate Strings(w2709) -> (w2710:string)
                n1812 = Concatenate Strings(w2718) -> (w2717:string)
                n1813 = Concatenate Strings(w2720) -> (w2713:string)
                n1814 = Equal?(x=w2713, y=w2717) -> (x = y?=w2708:bool)
                n1815 = Equal?(x=w2713, y=w2710) -> (x = y?=w2714:bool)
                n1816 = Or(x=w2708, y=w2714) -> (x .or. y?=→"x = y?":bool)
              }
            }
          }
        }
        n1817 = local read "x = y?"() -> (w2689:bool)
        n1818 = And(x="EDIT", y=w2689) -> (x .and. y?=w2687:bool)
        n1819 = case shown="True" w2687 {
          tunnel: [u8 2 ("Disabled") u8 0 ("Disabled")] -> w2686
          tunnel: [w2893 TRUE ("Visible")] -> w2685
          frame False {
            w2893 = FALSE ("Visible")
            n1820 = local write "EDIT 2"(w2893) -> ()
          }
          frame True {
          }
        }
        n1821 = case shown="True" "SAVE" {
          frame False {
          }
          frame True {
            n1822 = stacked-sequence {
              seq-local: [w2748 _ _] -> [_ w2889 _]
              frame #0 {
                w2744 = 0.0 ("number")
                w2745 = 0.0 ("number")
                (unwired) i16 5 ("precision (6)")
                # "[CH1]    - FF\n[CH2]   - TEMPERATURE\n[CH3]    - Humidity\n[CH4]    - AIR TEMP\n[CH5]\\- Visa Uno\n[CH6] \\- Visa Due\n[CH7]  \\- file path\n[CH8]   - Displacement Gain\n[CHA]   - Stroke Gain\n[CHB]   - Stroke PID Gain\n[CHC]   -Language Selection\n[CHD]   -Power +\n[CHE]   -Power_\n[CHF]   -Heater\n[CHG]   -Humidity Wet\n[CHH]   -Humidity Dry\n[CHI]   -Integral Time"
                n1823 = local read "Language Selection"() -> (w2791:enum16{"English", "Russian"})
                n1824 = Path To String(path="File Path") -> (string=w2807:string)
                n1825 = Number To Fractional String(number=w2744, width (-)=i16 10 ("precision (6)"), precision (6)=i16 5) -> (F-format string=w2798:string)  [unwired: 1 in]
                n1826 = Number To Fractional String(number=w2791, width (-)=i16 10 ("precision (6)"), precision (6)=i16 5) -> (F-format string=w2787:string)  [unwired: 1 in]
                n1827 = Number To Fractional String(number=w2745, width (-)=i16 10 ("precision (6)"), precision (6)=i16 5) -> (F-format string=w2781:string)  [unwired: 1 in]
                n1828 = Number To Fractional String(number=w2745, width (-)=i16 10 ("precision (6)"), precision (6)=i16 5) -> (F-format string=w2778:string)  [unwired: 1 in]
                n1829 = Number To Fractional String(number=w2745, width (-)=i16 10 ("precision (6)"), precision (6)=i16 5) -> (F-format string=w2773:string)  [unwired: 1 in]
                n1830 = Number To Fractional String(number=w2745, width (-)=i16 10 ("precision (6)"), precision (6)=i16 5) -> (F-format string=w2770:string)  [unwired: 1 in]
                n1831 = Number To Fractional String(number=w2745, width (-)=i16 10 ("precision (6)"), precision (6)=i16 5) -> (F-format string=w2765:string)  [unwired: 1 in]
                n1832 = local read "Com Port 1"() -> (w2747:refnum<visa-resource-name>)
                n1833 = local read "Com Port 2"() -> (w2746:refnum<visa-resource-name>)
                n1834 = Concatenate Strings(w2807, "\\" ("string")) -> (w2806:string)
                n1835 = Number To Fractional String(number=w2744, width (-)=i16 10 ("precision (6)"), precision (6)=i16 5) -> (F-format string=w2839:string)  [unwired: 1 in]
                n1836 = Number To Fractional String(number=w2744, width (-)=i16 10 ("precision (6)"), precision (6)=i16 5) -> (F-format string=w2838:string)  [unwired: 1 in]
                n1837 = Number To Fractional String(number=w2744, width (-)=i16 10 ("precision (6)"), precision (6)=i16 5) -> (F-format string=w2832:string)  [unwired: 1 in]
                n1838 = Number To Fractional String(number=w2744, width (-)=i16 10 ("precision (6)"), precision (6)=i16 5) -> (F-format string=w2826:string)  [unwired: 1 in]
                n1839 = Number To Fractional String(number=w2744, width (-)=i16 10 ("precision (6)"), precision (6)=i16 5) -> (F-format string=w2799:string)  [unwired: 1 in]
                n1840 = Concatenate Strings("[CHA]" ("string"), w2798, "- Stroke Gain" ("string"), "\r") -> (w2792:string)
                n1841 = Concatenate Strings("[CHC]" ("string"), w2787, "-Language Selection" ("string"), "\r") -> (w2784:string)
                n1842 = Concatenate Strings("[CHD]" ("string"), w2781, "-Power +" ("string"), "\r") -> (w2763:string)
                n1843 = Concatenate Strings("[CHG]" ("string"), w2770, "-Humidity Wet" ("string"), "\r") -> (w2760:string)
                n1844 = Concatenate Strings("[CHH]" ("string"), w2765, "-Humidity Dry" ("string"), "\r") -> (w2759:string)
                n1845 = Concatenate Strings("[CH1]" ("string"), w2839, " - FF" ("string"), "\r") -> (w2837:string)
                n1846 = Concatenate Strings("[CH2]" ("string"), w2838, " - TEMPERATURE" ("string"), "\r") -> (w2836:string)
                n1847 = Concatenate Strings("[CH3]" ("string"), w2832, " - Humidity" ("string"), "\r") -> (w2829:string)
                n1848 = Concatenate Strings("[CH4]" ("string"), w2826, " - AIR TEMP" ("string"), "\r") -> (w2822:string)
                n1849 = Concatenate Strings("[CH5]" ("string"), w2747, "- Visa Uno" ("string"), "\r") -> (w2815:string)
                n1850 = Concatenate Strings("[CH6]" ("string"), w2746, "- Visa Due" ("string"), "\r") -> (w2810:string)
                n1851 = Concatenate Strings("[CH7]" ("string"), w2806, "- file path" ("string"), "\r") -> (w2809:string)
                n1852 = Concatenate Strings("[CH8]" ("string"), w2799, "- Displacement Gain" ("string"), "\r") -> (w2802:string)
                n1853 = Concatenate Strings("[CHE]" ("string"), w2778, "-Power_" ("string"), "\r") -> (w2762:string)
                n1854 = Concatenate Strings("[CHF]" ("string"), w2773, "-Heater" ("string"), "\r") -> (w2761:string)
                n1855 = Concatenate Strings(w2837, w2836, w2829, w2822, w2815, w2810, w2809, w2802, w2792, w2784, w2763, w2762, w2761, w2760, w2759) -> (w2748:string)
                "gain" <- w2748
              }
              frame #1 {
                w2850 = 0.0 ("number")
                n1856 = local read "Camera Port :"() -> (w2853:string)
                n1857 = local read "C3 :"() -> (w2861:refnum<visa-resource-name>)
                n1858 = local read "Com Port 3"() -> (w2862:refnum<visa-resource-name>)
                n1859 = Concatenate Strings("[CH8]" ("string"), w2853, "- Visa Camera" ("string"), "\r") -> (w2852:string)
                n1860 = Concatenate Strings("[CH7]" ("string"), w2861, "- Visa Humidity" ("string"), "\r") -> (w2857:string)
                n1861 = Number To Fractional String(number=w2850, width (-)=i16 10 ("precision (6)"), precision (6)=i16 5) -> (F-format string=w2877:string)  [unwired: 1 in]
                n1862 = Concatenate Strings("[CHL]" ("string"), w2862, "- Visa humid" ("string"), "\r") -> (w2865:string)
                n1863 = Number To Fractional String(number=w2850, width (-)=i16 10 ("precision (6)"), precision (6)=i16 5) -> (F-format string=w2884:string)  [unwired: 1 in]
                n1864 = Concatenate Strings("[CHK]" ("string"), w2877, "-TEMP INTERCEPT" ("string"), "\r") -> (w2873:string)
                n1865 = Concatenate Strings("[SNO]" ("string"), "" ("string"), "-" ("string"), "\r") -> (w2870:string)
                n1866 = Concatenate Strings("[CHJ]" ("string"), w2884, "-AIR TEMP INTERCEPT" ("string"), "\r") -> (w2874:string)
                n1867 = String To Path(string="C:\\LAB-IQ\\calibrate WO 2465.dcf") -> (path=w2863:path)
                n1868 = Concatenate Strings(w2889, w2874, w2873, w2870, w2865, w2857, w2852) -> (w2888:string)
                n1869 = call <vilib>:"Write Characters To File.vi"("append to file? (new file:F)"=FALSE, "character string"=w2888, "file path (dialog if empty)"=w2863) -> ()  [unwired: 2 in, 1 out]
              }
              frame #2 {
                n1870 = local write "Lan flag"(0.0 ("Lan flag")) -> ()
                n1871 = local write "conststatus"(0.0 ("rpm value : 2")) -> ()
                n1872 = local write "SAVE"(FALSE ("OK Button 14")) -> ()
              }
            }
          }
        }
        n1873 = property on="EDIT 2" class="Bool (strict)"("Visible"=w2685) -> ()  [unwired: 2 in, 2 out]
        n1874 = property on="SAVE" class="Bool (strict)"("Visible"=w2685) -> ()  [unwired: 2 in, 2 out]
        n1875 = property on="visa due" class="CmbBox"("Disabled"=w2686) -> ()  [unwired: 2 in, 2 out]
        n1876 = property on="File Path" class="Path"("Disabled"=w2686) -> ()  [unwired: 2 in, 2 out]
        n1877 = property on="Language Selection" class="Enum (strict)"("Visible"=w2685) -> ()  [unwired: 2 in, 2 out]
        n1878 = property on="SPEED OUT:" class="DigNum (strict)"("Disabled"=w2686) -> ()  [unwired: 2 in, 2 out]
      }
    }
    n1879 = local read "RUN"() -> (w2212:bool)
    n1880 = local read "RUN"() -> (w2210:bool)
    n1881 = case shown="True" "EDIT 3" {
      frame False {
      }
      frame True {
        n1882 = local write "EDIT 3"(FALSE ("EDIT 3")) -> ()
        n1883 = local write "Main Tab"(T2."About" ("Main Tab")) -> ()
      }
    }
    n1884 = case shown="False" w2212 {
      frame False {
        n1885 = local read "stopT"() -> (w2900:bool)
